vi "macro_Ramsete_Execute.vi"   [LabVIEW 2019, in "Trajectory_Library.lvlib"]
uses:
  ProfiledPIDController_NewPeriod.vi
  PIDController_NewPeriod.vi
  TrapProfState_New.vi
  <vilib>/Rock Robotics/SystemInterfaces/NetworkCommunication/NetComm_UsageReport_report.vi
  Util_LibraryGlobals.vi
  Trajectory_Library.lvlib
types:
  T1 = typedef "Trajectory_Library.lvlib/RAMSETE_EXE_TUNING.ctl" = cluster{"B":dbl, "Zeta":dbl, "X Tolerance M":dbl, "Y Tolerance M":dbl, "Heading Tolerance RAD":dbl, "Track Width M":dbl, "Max Speed M/S":dbl}
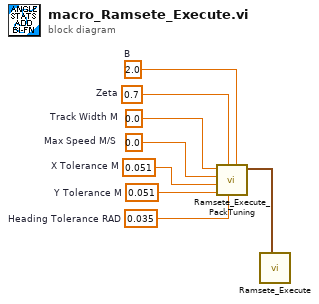
[diagram p0: block diagram]
diagram:
  w1 = 0.0  # Track Width M
  w2 = 0.0  # Max Speed M/S
  w3 = 0.051  # X Tolerance M
  w4 = 0.051  # Y Tolerance M
  w5 = 0.7  # Zeta
  w6 = 0.035  # Heading Tolerance RAD
  w7 = 2.0  # B
  n1 = call "Ramsete_Execute_PackTuning.vi"("B"=w7, "Heading Tolerance RAD"=w6, "Zeta"=w5, "Y Tolerance M"=w4, "X Tolerance M"=w3, "Max Speed M/S"=w2, "Track Width M"=w1) -> ("RAMSETE_EXE_TUNING"=w8:T1)  [unwired: 4 in]
  n2 = call "Ramsete_Execute.vi"("RAMSETE_EXE_TUNING"=w8) -> ()  [unwired: 6 in, 5 out]
